vi "SMO.TimedLoop.GetSetpoint.vi"(8 "error in (no error)":errorcluster, 11 "SMO.TimedLoop":refnum<class "SMO.TimedLoop.lvclass">) -> (0 "error out":errorcluster, 2 "Setpoint":dbl, 3 "SMO.TimedLoop out":refnum<class "SMO.TimedLoop.lvclass">)   [LabVIEW 2013, in "SMO.TimedLoop.lvclass"]
doc: "---------------------------------------------------------------\nJKI State Machine Objects™\nhttp://jki.net/state-machine-objects/\nCopyright (C) 2005-2015, JKI <info@jki.net>\nALL RIGHTS RESERVEDJKI State Machine Objects (SMO) 1.0.0.5\nJKI - JKI\nCopyright (c) 2016, JKI"
uses:
  SMO.TimedLoop.lvclass
  SMO.TimedLoop.lvclass/SMO.TimedLoop.ctl
panel:
  # "For instructions on how to use the JKI State Machine Objects, examples and video tutorials, visit:\nhttp://jki.net/state-machine-objects/\n\nJKI State Machine Objects™\nhttp://jki.net/state-machine-objects/\nCopyright (C) 2005-2015, JKI <info@jki.net>\nALL RIGHTS RESERVED"
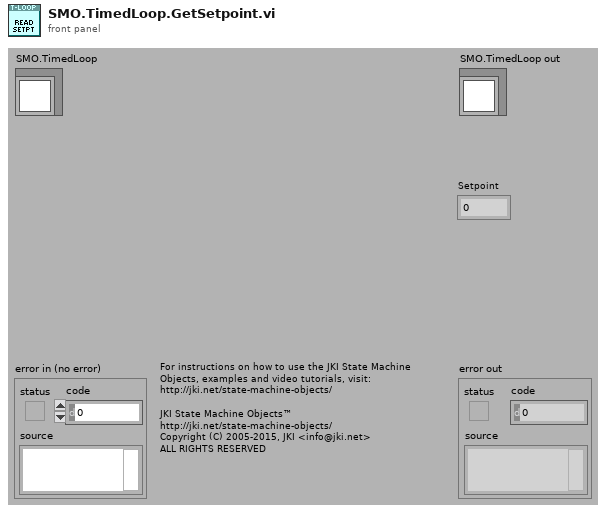
[diagram p1: front panel]
types:
  T1 = typedef "SMO.TimedLoop.lvclass/PrivateData--Ref.ctl" = refnum<data-value>
  T2 = typedef "SMO.TimedLoop.lvclass/PrivateData--Cluster.ctl" = cluster{"Public Events":T3, "Setpoint":T4, "Private Events":T5}
  T3 = typedef "SMO.TimedLoop.lvclass/PublicEvents--Cluster.ctl" = cluster{"Setpoint Changed":refnum<user-event>, "Value Changed":refnum<user-event>}
  T4 = typedef "SMO.TimedLoop.lvclass/Data.ctl" = dbl
  T5 = typedef "SMO.TimedLoop.lvclass/PrivateEvents--Cluster.ctl" = cluster{"AsyncMethod":refnum<user-event>}
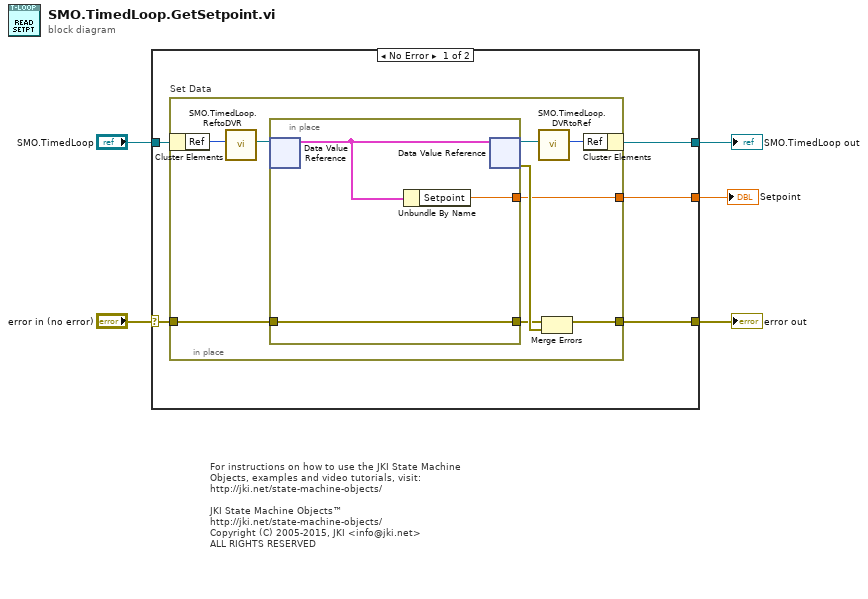
[diagram p0: block diagram]
diagram:
  # "For instructions on how to use the JKI State Machine Objects, examples and video tutorials, visit:\nhttp://jki.net/state-machine-objects/\n\nJKI State Machine Objects™\nhttp://jki.net/state-machine-objects/\nCopyright (C) 2005-2015, JKI <info@jki.net>\nALL RIGHTS RESERVED"
  n1 = case shown="No Error" "error in (no error)" {
    selector: "error in (no error)" -> [w9 w23]
    tunnel: "SMO.TimedLoop" -> [w10 w24]
    tunnel: [w8 w23] -> w4
    tunnel: [w7 w24] -> w3
    tunnel: [w6 _] -> w1
    frame No Error {
      n2 = in-place "Set Data" {
        in-place-border: w9 -> [w19]
        in-place-border: [w16] -> w8
        in-place-border: [w11] -> w6
        n3 = in-place-cluster #1(w10) -> ("Ref"=w15:u32)
        n4 = call "SMO.TimedLoop.ReftoDVR.vi"("Ref"=w15) -> ("Ref"=w14:T1)  [unwired: 10 in]
        n5 = in-place {
          in-place-border: w19 -> [w22]
          in-place-border: [w22] -> w17
          in-place-border: [w21] -> w11
          n6 = in-place-dvr #2(w14) -> (w20:T2)  [unwired: 1 out]
          n7 = Unbundle By Name(w20) -> ("Setpoint"=w21:T4)
          n8 = in-place-dvr #2(w20) -> (w13:T1, w18:errorcluster)
        }
        n9 = call "SMO.TimedLoop.DVRtoRef.vi"("Ref"=w13) -> ("Ref"=w12:u32)  [unwired: 10 in]
        n10 = Merge Errors(w17, w18) -> (w16:errorcluster)
        n11 = in-place-cluster #1("Ref"=w12) -> (w7:refnum<class "SMO.TimedLoop.lvclass">)
      }
    }
    frame Error {
    }
  }
  "error out" <- w4
  "SMO.TimedLoop out" <- w3
  "Setpoint" <- w1
